vi "PV ActiveLine miscellaneous.vi"(8 "error in (no error)":errorcluster, 9 "PV ActiveLine miscellaneous - Cluster":T1={"Parameter"=enum." Keyboard interlock (008)", "Parameter\nread only<->describe"=FALSE, "off<->on   "=TRUE, "Unit adress"=10} {"Unit adress" min=1 max=255 step=1}, 10 "Adress of unit":u16=10 max=999 step=1, 11 "VISA session":refnum<visa-resource-name>) -> (0 "error out":errorcluster, 2 "response (data)":string, 3 "dup VISA session":refnum<visa-resource-name>)   [LabVIEW 2021, in "Pfeiffer Vacuum.lvlib"]
doc: "There are 4 parameters available, only one of which can be enabled at a time. \n\nKeyboard interlock (008)\nUnit adress (797)\nOperating hours (314)\nHardware version (354)\n\nNote: Any settings for an parameter that is not selected will be ignored. If a value is out of range, it will be changed to either the upper or the lower limit of the range."
uses:
  <instrlib>/Pfeiffer Vacuum/Pfeiffer Vacuum.lvlib
  <instrlib>/Pfeiffer Vacuum/Public/ActiveLine/PV ActiveLine miscellaneous - Cluster.ctl
panel:
  # "<------------  -----------> \n Keyboard interlock :             OFF                          ON"
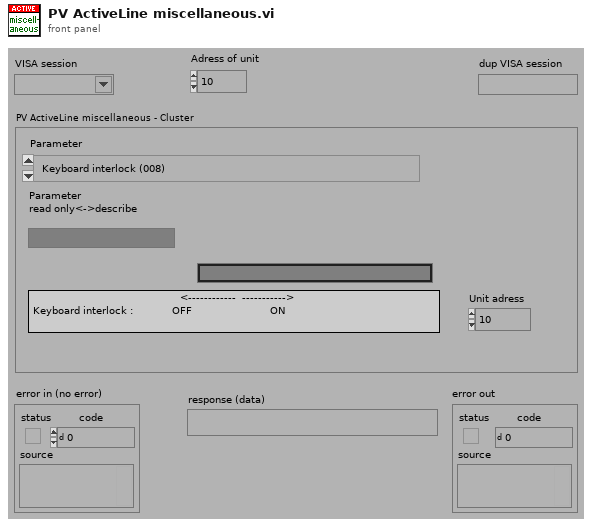
[diagram p1: front panel]
types:
  T1 = typedef "Pfeiffer Vacuum.lvlib/PV ActiveLine miscellaneous - Cluster.ctl" = cluster{"Parameter":enum16{" Keyboard interlock (008)", " Unit adress (797)", " Operating hours TPG36x (314)", " Hardware Version (354)"}, "Parameter\nread only<->describe":bool, "off<->on   ":bool, "Unit adress":i16}
  T2 = enum16{" Keyboard interlock (008)", " Unit adress (797)", " Operating hours TPG36x (314)", " Hardware Version (354)"}
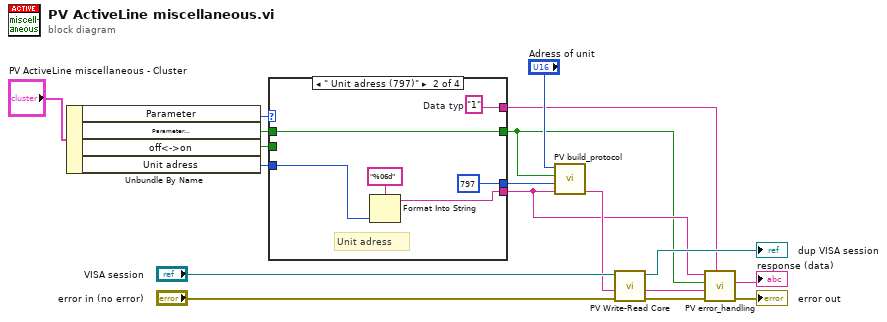
[diagram p0: block diagram]
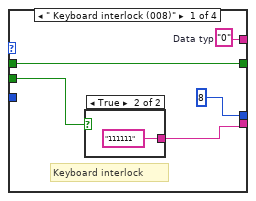
[diagram p2: hidden frame]
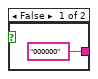
[diagram p3: hidden frame]
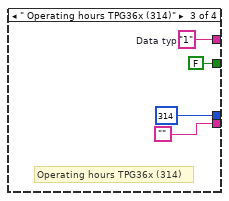
[diagram p4: hidden frame]
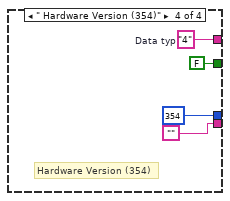
[diagram p5: hidden frame]
diagram:
  n1 = Unbundle By Name("PV ActiveLine miscellaneous - Cluster") -> ("Parameter"=w16:T2, "Parameter\nread only<->describe"=w15:bool, "off<->on"=w13:bool, "Unit adress"=w12:i16)
  n2 = case shown="\" Unit adress (797)\"" w16 {
    tunnel: [u16 8 ("Parameter-number") u16 797 ("Parameter-number") u16 314 ("Parameter-number") u16 354 ("Parameter-number")] -> w17
    tunnel: [w19 w30 "" ""] -> w4
    tunnel: [w21 w28 FALSE ("Parameter\nread only<->describe") FALSE ("Parameter\nread only<->describe")] -> w3
    tunnel: w15 -> [w21 w28 _ _]
    tunnel: w13 -> [w20 _ _ _]
    tunnel: w12 -> [_ w27 _ _]
    tunnel: [w22 w26 w34 w38] -> w5
    frame " Keyboard interlock (008)" {
      w22 = "0"  # Data typ
      # "Keyboard interlock"
      n3 = case shown="True" w20 {
        tunnel: ["000000" ("Data") "111111" ("Data")] -> w19
        frame False {
        }
        frame True {
        }
      }
    }
    frame " Unit adress (797)" {
      w26 = "1"  # Data typ
      # "Unit adress"
      n4 = Format Into String(format string="%06d" ("Format-String"), w27) -> (resulting string=w30:string)  [unwired: 2 in, 1 out]
    }
    frame " Operating hours TPG36x (314)" {
      w34 = "1"  # Data typ
      # "Operating hours TPG36x (314)"
    }
    frame " Hardware Version (354)" {
      w38 = "4"  # Data typ
      # "Hardware Version (354)"
    }
  }
  n5 = call <instrlib>:"PV build_protocol.vi"("Data"=w4, "Parameter-number"=w17, "parameter\nread<->describe"=w3, "Adress"="Adress of unit") -> ("output"=w9:string)  [unwired: 3 in]
  n6 = call <instrlib>:"PV Write-Read Core.vi"("error in"="error in (no error)", "Write data in"=w9, "VISA session"="VISA session") -> ("error out"=w6:errorcluster, "response (data) out"=w7:string, "dup VISA session"=→"dup VISA session":refnum<visa-resource-name>)  [unwired: 2 in]
  n7 = call <instrlib>:"PV error_handling.vi"("Data Typ in"=w5, "error in"=w6, "response (data) in"=w7, "Parameter\nread only<->describe"=w3, "data in"=w4) -> ("error out"=→"error out":errorcluster, "Data out"=→"response (data)":string)  [unwired: 4 in, 1 out]
